vi "INIT_Prueba.vi"(8 "error in (no error)":errorcluster, 10 "dup Message Queue":refnum<queue>, 11 "Prueba33 in":refnum<class "Prueba33.lvclass">) -> (0 "error out":errorcluster, 3 "Prueba33 out":refnum<class "Prueba33.lvclass">)   [LabVIEW 2019, in "Prueba33.lvclass"]
uses:
  Prueba33.lvclass
  QMH/Message Queue/Message Cluster.ctl
  Controles/Tab.ctl
  Prueba33.lvclass/Prueba33.ctl
  RerenceAllControlsToolkit/_get control reference by name.vi
  QMH/Message Queue/Enqueue Message (Single).vi
  QMH/Message Queue/Message Queue.lvlib
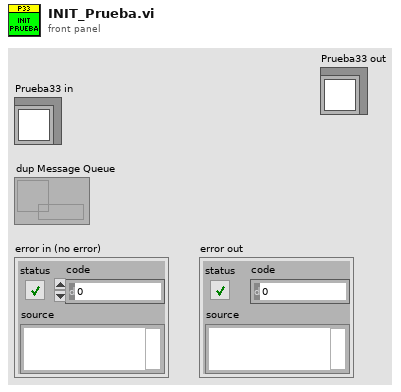
[diagram p1: front panel]
types:
  T1 = typedef "Prueba33.lvclass/Tab.ctl" = enum32{"Main", "D1_A", "D1_B", "D2_A", "D2_B", "D3_A", "D3_B", "D4_A", "D4_B"}
  T2 = cluster{"ControlName":string, "ControlReference":refnum<vi>}[]
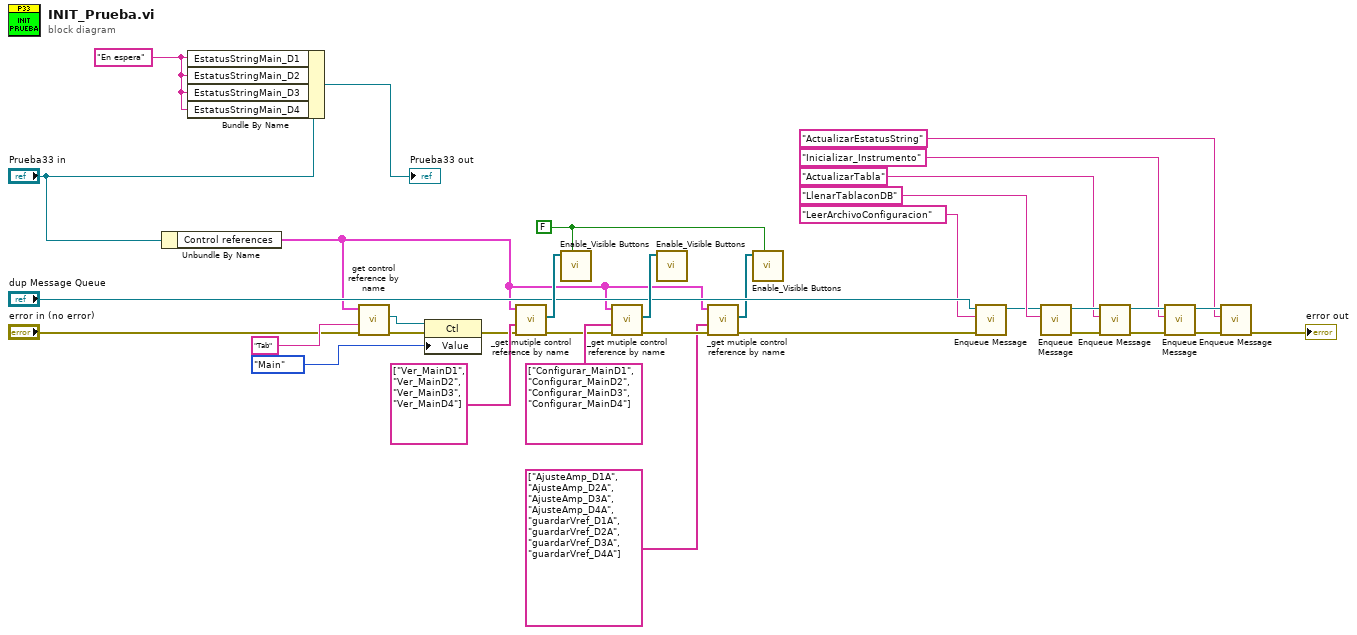
[diagram p0: block diagram]
diagram:
  w8 = "En espera" ("Message")
  w1 = FALSE ("Enable? (T)")
  n1 = Unbundle By Name("Prueba33 in") -> ("Control references"=w6:T2)
  n2 = Bundle By Name(cluster="Prueba33 in", "EstatusStringMain_D1"=w8, "EstatusStringMain_D2"=w8, "EstatusStringMain_D3"=w8, "EstatusStringMain_D4"=w8) -> (→"Prueba33 out":refnum<class "Prueba33.lvclass">)
  n3 = call-poly "get control reference by name.vi"("error in (no error)"="error in (no error)", "Control name"="Tab", "Control references"=w6) -> ("error out"=w26:errorcluster, "Ctl Refnum"=w25:refnum<vi>)  [unwired: 3 in]
  n4 = property class="Ctl"(reference=w25, error in=w26, "Value"=Tab."Main" ("Tab")) -> (error out=w30:errorcluster)  [unwired: 1 out]
  n5 = call "_get mutiple control reference by name.vi"("error in (no error)"=w30, "Control names"=string[] ["Ver_MainD1", "Ver_MainD2", "Ver_MainD3", "Ver_MainD4"], "Control references"=w6) -> ("error out"=w5:errorcluster, "References"=w32:refnum<vi>[])  [unwired: 3 in]
  n6 = call "Enable_Visible Buttons.vi"("Enable? (T)"=w1, "Controls Ref Array"=w32) -> ()  [unwired: 10 in]
  n7 = call "_get mutiple control reference by name.vi"("error in (no error)"=w5, "Control names"=string[] ["Configurar_MainD1", "Configurar_MainD2", "Configurar_MainD3", "Configurar_MainD4"], "Control references"=w6) -> ("error out"=w4:errorcluster, "References"=w33:refnum<vi>[])  [unwired: 3 in]
  n8 = call "Enable_Visible Buttons.vi"("Controls Ref Array"=w33) -> ()  [unwired: 11 in]
  n9 = call "_get mutiple control reference by name.vi"("error in (no error)"=w4, "Control names"=string[] ["AjusteAmp_D1A", "AjusteAmp_D2A", "AjusteAmp_D3A", "AjusteAmp_D4A", "guardarVref_D1A", "guardarVref_D2A", "guardarVref_D3A", "guardarVref_D4A"], "Control references"=w6) -> ("error out"=w3:errorcluster, "References"=w7:refnum<vi>[])  [unwired: 3 in]
  n10 = call "Enable_Visible Buttons.vi"("Enable? (T)"=w1, "Controls Ref Array"=w7) -> ()  [unwired: 10 in]
  n11 = call-poly "Enqueue Message.vi"("error in (no error)"=w3, "Message"="LeerArchivoConfiguracion", "Message Queue"="dup Message Queue") -> ("dup Message Queue"=w22:refnum<queue>)  [unwired: 7 in, 1 out]
  n12 = call-poly "Enqueue Message.vi"("Message"="LlenarTablaconDB", "Message Queue"=w22) -> ("error out"=w19:errorcluster, "dup Message Queue"=w18:refnum<queue>)  [unwired: 8 in]
  n13 = call-poly "Enqueue Message.vi"("error in (no error)"=w19, "Message"="ActualizarTabla", "Message Queue"=w18) -> ("error out"=w15:errorcluster, "dup Message Queue"=w20:refnum<queue>)  [unwired: 7 in]
  n14 = call-poly "Enqueue Message.vi"("error in (no error)"=w15, "Message"="Inicializar_Instrumento", "Message Queue"=w20) -> ("error out"=w14:errorcluster, "dup Message Queue"=w13:refnum<queue>)  [unwired: 7 in]
  n15 = call-poly "Enqueue Message.vi"("error in (no error)"=w14, "Message"="ActualizarEstatusString", "Message Queue"=w13) -> ("error out"=→"error out":errorcluster)  [unwired: 7 in, 1 out]
